vi "reset.vi"(8 "error in (no error)":errorcluster, 11 "DL090624AnalyserScaffold in":refnum<class "AnalyserDL090624Scaffold.lvclass">) -> (0 "error out":errorcluster, 3 "DL090624AnalyserScaffold out":refnum<class "AnalyserDL090624Scaffold.lvclass">)   [LabVIEW 2010, in "AnalyserDL090624Scaffold.lvclass"]
uses:
  AnalyserDL090624Scaffold.lvclass
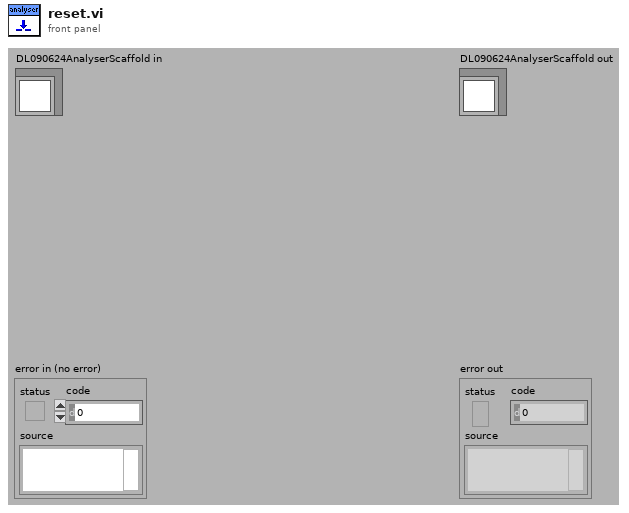
[diagram p1: front panel]
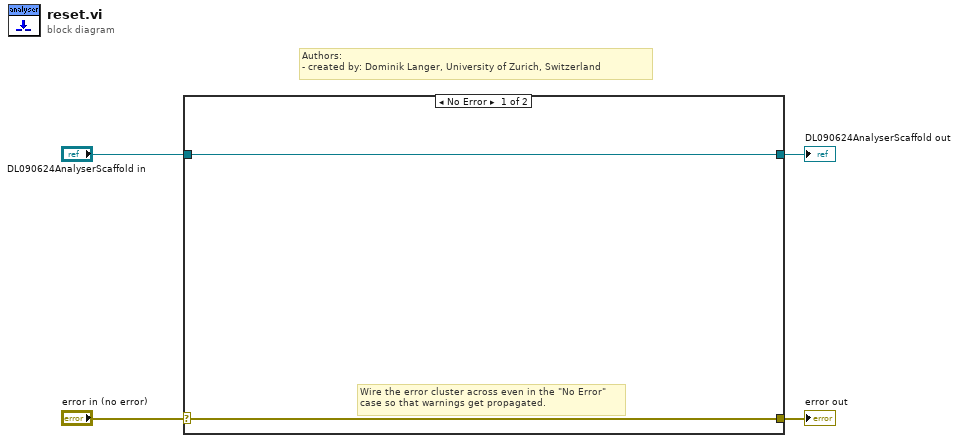
[diagram p0: block diagram]
diagram:
  # "Authors: \n- created by: Dominik Langer, University of Zurich, Switzerland"
  n1 = case shown="No Error" "error in (no error)" {
    selector: "error in (no error)" -> [w5 w8]
    tunnel: [w5 w8] -> w3
    tunnel: [w6 w7] -> w1
    tunnel: "DL090624AnalyserScaffold in" -> [w6 w7]
    frame No Error {
      # "Wire the error cluster across even in the \"No Error\"\ncase so that warnings get propagated."
    }
    frame Error {
    }
  }
  "error out" <- w3
  "DL090624AnalyserScaffold out" <- w1
